vi "PCE-Offset.vi"(0 "connection ID":refnum<k5>, 1 "DEC":dbl=3.0 min=3.0 max=1800.0 step=1.0, 2 "RA":dbl=3.0 min=3.0 max=1800.0 step=1.0, 11 "error in":errorcluster) -> (4 "connection ID dup":refnum<k5>, 15 "error out":errorcluster)   [LabVIEW 2011]
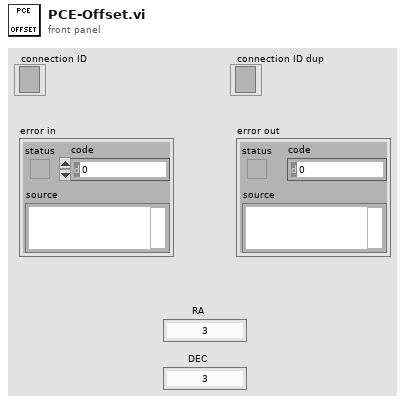
[diagram p1: front panel]
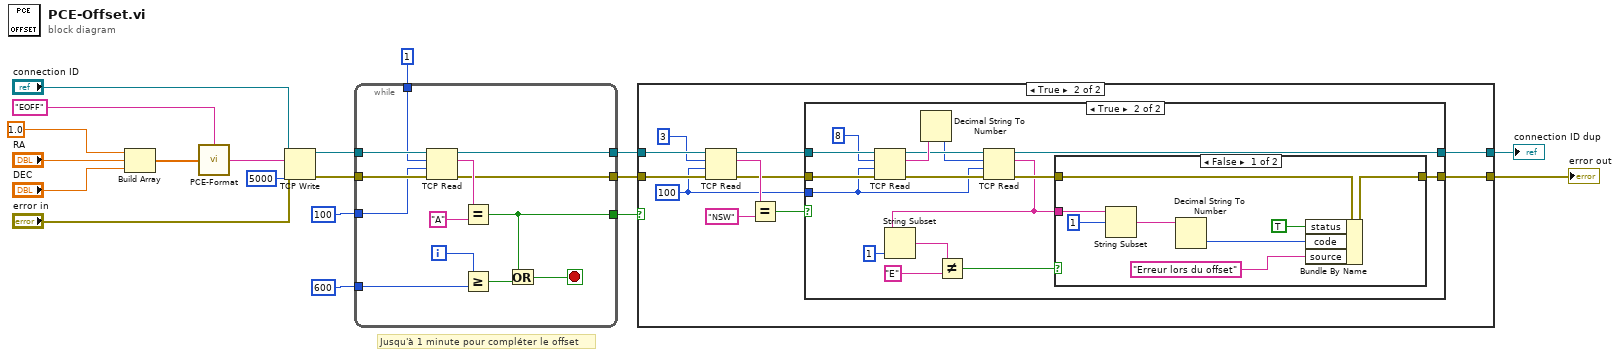
[diagram p0: block diagram]
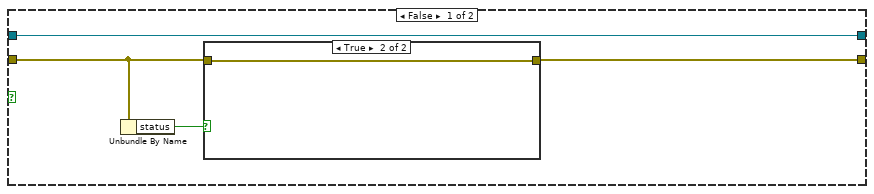
[diagram p2: hidden frame]
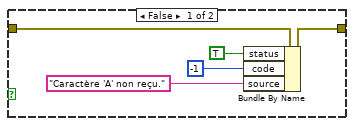
[diagram p3: hidden frame]
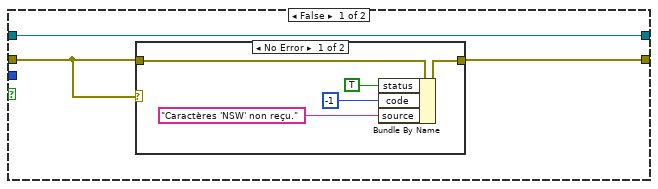
[diagram p4: hidden frame]
diagram:
  # "Jusqu'à 1 minute pour compléter le offset"
  n1 = Build Array(1.0 ("RA"), "RA", "DEC") -> (w16:dbl[])
  n2 = call "PCE-Format.vi"("Commande"="EOFF", "Arguments"=w16) -> ("Chaîne formatée"=w14:string)  [unwired: 13 in]
  n3 = TCP Write(connection ID="connection ID", data in=w14, error in (no error)="error in", 9:5000 ("timeout ms (25000)")) -> (connection ID out=w7:refnum<k5>, error out=w6:errorcluster)  [unwired: 1 out]
  n4 = while {
    tunnel: w6 -> [w31]
    tunnel: w7 -> [w32]
    tunnel: [w26] -> w4
    tunnel: [w25] -> w5
    tunnel: [w23] -> w1
    tunnel: 100 ("timeout ms (25000)") -> [w22]
    tunnel: 1 ("bytes to read") -> [w21]
    tunnel: 600 ("y") -> [w20]
    i -> [w30]
    stop <- w24 stop-if-true
    n5 = TCP Read(connection ID=w32, bytes to read=w21, error in (no error)=w31, 9:w22) -> (connection ID out=w25:refnum<k5>, data out=w29:string, error out=w26:errorcluster)  [unwired: 1 in]
    n6 = Equal?(x=w29, y="A") -> (x = y?=w23:bool)
    n7 = Greater Or Equal?(x=w30, y=w20) -> (x >= y?=w27:bool)
    n8 = Or(x=w23, y=w27) -> (x .or. y?=w24:bool)
  }
  n9 = case shown="True" w1 {
    tunnel: w4 -> [w34 w52]
    tunnel: w5 -> [w36 w53]
    tunnel: [w33 w44] -> w2
    tunnel: [w36 w43] -> w3
    frame False {
      n10 = Unbundle By Name(w34) -> ("status"=w35:bool)
      n11 = case shown="True" w35 {
        tunnel: w34 -> [w40 w42]
        tunnel: [w39 w42] -> w33
        frame False {
          n12 = Bundle By Name(cluster=w40, "status"=TRUE, "code"=-1, "source"="Caractère 'A' non reçu.") -> (w39:errorcluster)
        }
        frame True {
        }
      }
    }
    frame True {
      w45 = 100 ("timeout ms (25000)")
      n13 = TCP Read(connection ID=w53, bytes to read=3, error in (no error)=w52, 9:w45) -> (connection ID out=w47:refnum<k5>, data out=w50:string, error out=w46:errorcluster)  [unwired: 1 in]
      n14 = Equal?(x=w50, y="NSW") -> (x = y?=w48:bool)
      n15 = case shown="True" w48 {
        tunnel: w47 -> [w56 w78]
        tunnel: w46 -> [w54 w77]
        tunnel: w45 -> [_ w71]
        tunnel: [w55 w65] -> w44
        tunnel: [w56 w70] -> w43
        frame False {
          n16 = case shown="No Error" w54 {
            tunnel: w54 -> [w60 w62]
            tunnel: [w59 w62] -> w55
            frame No Error {
              n17 = Bundle By Name(cluster=w60, "status"=TRUE, "code"=-1, "source"="Caractères 'NSW' non reçu.") -> (w59:errorcluster)
            }
            frame Error {
            }
          }
        }
        frame True {
          n18 = TCP Read(connection ID=w78, bytes to read=8, error in (no error)=w77, 9:w71) -> (connection ID out=w74:refnum<k5>, data out=w75:string, error out=w73:errorcluster)  [unwired: 1 in]
          n19 = Decimal String To Number(string=w75) -> (number=w72:i32)  [unwired: 2 in, 1 out]
          n20 = TCP Read(connection ID=w74, bytes to read=w72, error in (no error)=w73, 9:w71) -> (connection ID out=w70:refnum<k5>, data out=w64:string, error out=w66:errorcluster)  [unwired: 1 in]
          n21 = String Subset(string=w64, length (rest)=1 ("length (rest)")) -> (substring=w67:string)  [unwired: 1 in]
          n22 = Not Equal?(x=w67, y="E") -> (x != y?=w63:bool)
          n23 = case shown="False" w63 {
            tunnel: [w83 w87] -> w65
            tunnel: w66 -> [w84 w87]
            tunnel: w64 -> [w82 _]
            frame False {
              n24 = String Subset(string=w82, offset (0)=1 ("length (rest)")) -> (substring=w80:string)  [unwired: 1 in]
              n25 = Decimal String To Number(string=w80) -> (number=w79:i32)  [unwired: 2 in, 1 out]
              n26 = Bundle By Name(cluster=w84, "status"=TRUE, "code"=w79, "source"="Erreur lors du offset") -> (w83:errorcluster)
            }
            frame True {
            }
          }
        }
      }
    }
  }
  "connection ID dup" <- w3
  "error out" <- w2
